vi "Init.vi"(8 "error in (no error)":errorcluster, 10 "Variant":variant, 11 "NKT in":refnum<class "NKT_Extreme.lvclass">) -> (0 "error out":errorcluster, 3 "NKT out":refnum<class "NKT_Extreme.lvclass">)   [LabVIEW 2020, in "NKT_Extreme.lvclass"]
uses:
  <instrlib>/Classes/Laser/NKT/NKT_Extreme.lvclass
  <instrlib>/NKTP_API/NKTP_API.lvlib
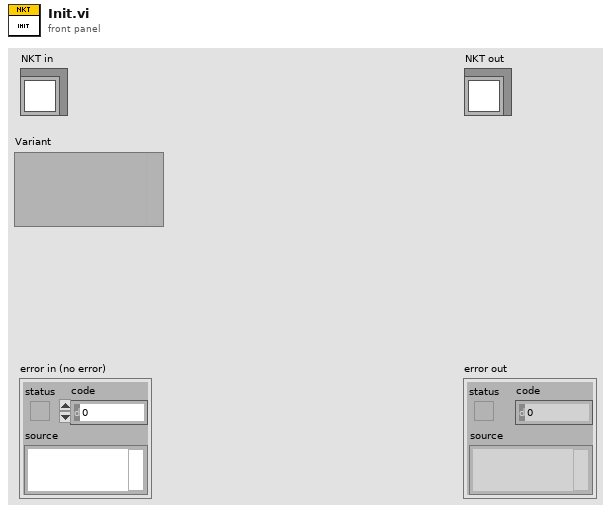
[diagram p1: front panel]
types:
  T1 = cluster{"Com":refnum<visa-resource-name>, "ID Laser":u8, "ID Split":u8, "ID RF":u8, "ID Select":u8, "ID Dummy":u8, "ID Dummy 2":u8}
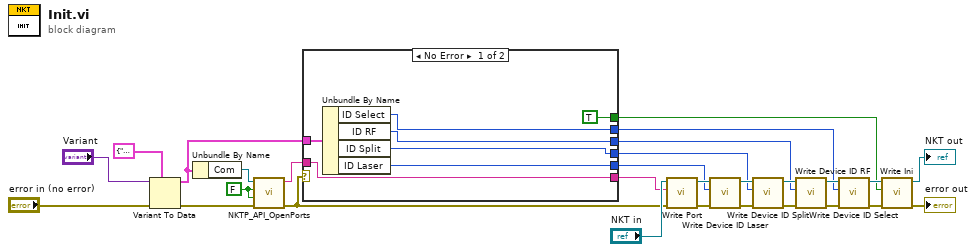
[diagram p0: block diagram]
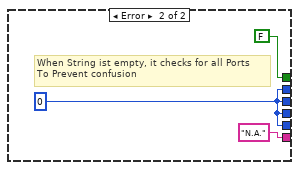
[diagram p2: hidden frame]
diagram:
  w24 = FALSE ("autoMode")
  n1 = Variant To Data(error in="error in (no error)", type=T1 {"Com"="", "ID Laser"=0, "ID Split"=0, "ID RF"=0, "ID Select"=0, "ID Dummy"=0, "ID Dummy 2"=0} ("input cluster"), Variant="Variant") -> (data=w8:T1, error out=w23:errorcluster)
  n2 = Unbundle By Name(w8) -> ("Com"=w25:refnum<visa-resource-name>)
  n3 = call <instrlib>:"NKTP_API_OpenPorts.vi"("error in"=w23, "liveMode"=w24, "autoMode"=w24, "portnames"=w25) -> ("error out"=w9:errorcluster, "portnames out"=w2:string)  [unwired: 6 in]
  n4 = case shown="No Error" w9 {
    tunnel: w8 -> [w35 _]
    tunnel: [w34 w37] -> w7
    tunnel: [w33 w37] -> w6
    tunnel: [w32 w37] -> w5
    tunnel: [w31 w37] -> w4
    tunnel: [TRUE ("Init") FALSE ("Init")] -> w3
    tunnel: [w29 "N.A." ("portnames out")] -> w1
    tunnel: w2 -> [w29 _]
    frame No Error {
      n5 = Unbundle By Name(w35) -> ("ID Select"=w34:u8, "ID RF"=w33:u8, "ID Split"=w32:u8, "ID Laser"=w31:u8)
    }
    frame Error {
      w37 = u8 0 ("ID Laser")
      # "When String ist empty, it checks for all Ports\nTo Prevent confusion"
    }
  }
  n6 = call-dynamic "Write Port.vi"("error in (no error)"=w9, "Port"=w1, "NKT in"="NKT in") -> ("error out"=w21:errorcluster, "NKT out"=w20:refnum<class "NKT_Extreme.lvclass">)  [unwired: 7 in]
  n7 = call-dynamic "Write Device ID Laser.vi"("error in (no error)"=w21, "Device ID Laser"=w4, "NKT in"=w20) -> ("error out"=w19:errorcluster, "NKT out"=w18:refnum<class "NKT_Extreme.lvclass">)  [unwired: 7 in]
  n8 = call-dynamic "Write Device ID Split.vi"("error in (no error)"=w19, "Device ID Split"=w5, "NKT in"=w18) -> ("error out"=w17:errorcluster, "NKT out"=w16:refnum<class "NKT_Extreme.lvclass">)  [unwired: 7 in]
  n9 = call-dynamic "Write Device ID RF.vi"("error in (no error)"=w17, "Device ID RF"=w6, "NKT in"=w16) -> ("error out"=w15:errorcluster, "NKT out"=w14:refnum<class "NKT_Extreme.lvclass">)  [unwired: 7 in]
  n10 = call-dynamic "Write Device ID Select.vi"("error in (no error)"=w15, "Device ID Select"=w7, "NKT in"=w14) -> ("error out"=w13:errorcluster, "NKT out"=w12:refnum<class "NKT_Extreme.lvclass">)  [unwired: 7 in]
  n11 = call-dynamic "Write Ini.vi"("error in (no error)"=w13, "Init"=w3, "NKT in"=w12) -> ("error out"=→"error out":errorcluster, "NKT out"=→"NKT out":refnum<class "NKT_Extreme.lvclass">)  [unwired: 7 in]
